vi "Set Desired Range.vi"(8 "error in (no error)":errorcluster, 10 "Desired Range":dbl format="%.3g", 11 "MWWL Verification in":refnum<class "MWWL Verification.lvclass">) -> (0 "error out":errorcluster, 3 "MWWL Verification out":refnum<class "MWWL Verification.lvclass">)   [LabVIEW 2018, in "MWWL Verification.lvlib" / "MWWL Verification.lvclass"]
uses:
  MWWL Verification.lvclass
  MWWL Verification.lvclass/MWWL Verification.ctl
  Range Controller Actor/Range Controller Actor Messages/Set Desired Range Msg/Set Desired Range Msg.lvclass
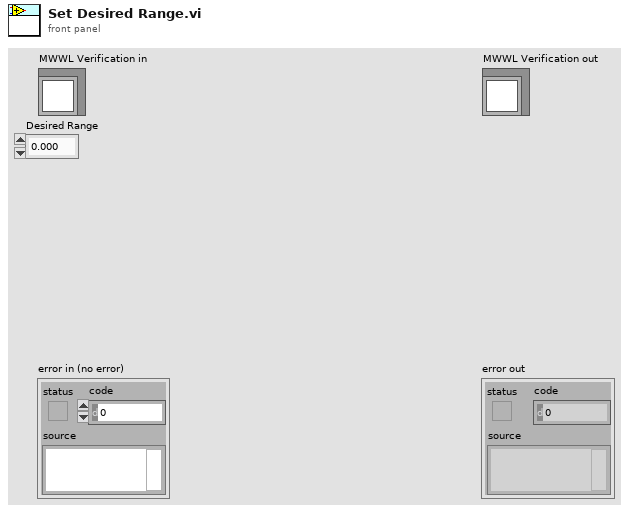
[diagram p1: front panel]
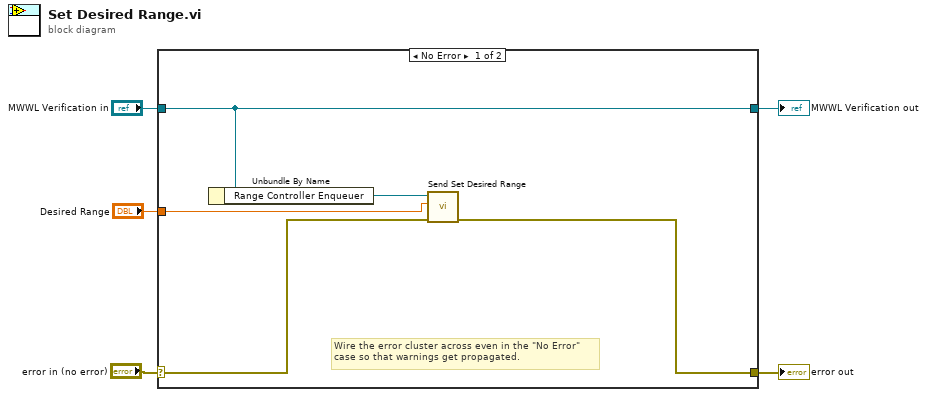
[diagram p0: block diagram]
diagram:
  n1 = case shown="No Error" "error in (no error)" {
    selector: "error in (no error)" -> [w7 w12]
    tunnel: [w6 w12] -> w4
    tunnel: [w10 w11] -> w2
    tunnel: "MWWL Verification in" -> [w10 w11]
    tunnel: "Desired Range" -> [w8 _]
    frame No Error {
      # "Wire the error cluster across even in the \"No Error\"\ncase so that warnings get propagated."
      n2 = Unbundle By Name(w10) -> ("Range Controller Enqueuer"=w9:refnum<class "Message Enqueuer.lvclass">)
      n3 = call "Send Set Desired Range.vi"("error in (no error)"=w7, "Desired Range"=w8, "Message Enqueuer in"=w9) -> ("error out"=w6:errorcluster)  [unwired: 7 in, 1 out]
    }
    frame Error {
    }
  }
  "error out" <- w4
  "MWWL Verification out" <- w2
